vi "Required Buffer Sizes.vi"(8 "error in (no error)":errorcluster, 11 "Transfer Configuration in":refnum<class "Transfer Configuration.lvclass">) -> (0 "error out":errorcluster, 1 "string size":u64 format="%d bytes", 2 "engine size":u64 format="%d bytes", 3 "Transfer Configuration out":refnum<class "Transfer Configuration.lvclass">)   [LabVIEW 2021, in "DSF Core.lvlib" / "Transfer Configuration.lvclass"]
uses:
  Transfer Configuration.lvclass
  Transfer Configuration.lvclass/Transfer Configuration.ctl
  Framework/Framework.lvclass
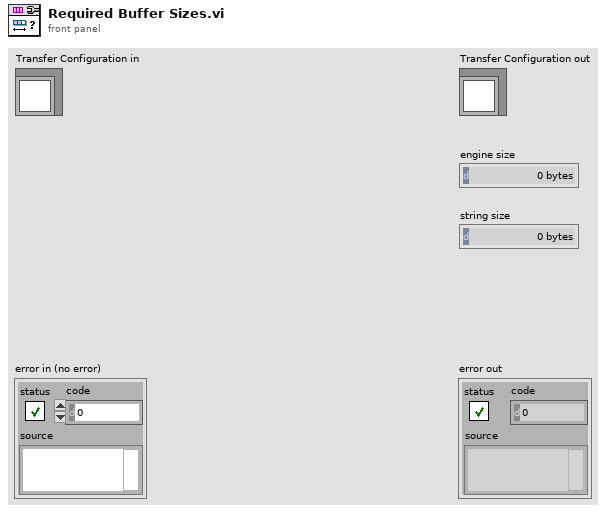
[diagram p1: front panel]
types:
  T1 = typedef "DSF Core.lvlib/Transfer Configuration.lvclass/Channel Configuration.ctl" = cluster{"configuration":T2, "component settings":T4[]}
  T2 = typedef "DSF Core.lvlib/Channel Configuration.lvclass/Core Channel Configuration.ctl" = cluster{"name":string, "units":string, "engine data type":T3, "string data type":T3, "string offset":u64}
  T3 = typedef "DSF Core.lvlib/DSF Data Type.ctl" = enum8{"Bool", "SGL", "DBL", "I8", "I16", "I32", "I64", "U8", "U16", "U32", "U64"}
  T4 = typedef "DSF Core.lvlib/DSF Settings Info.ctl" = cluster{"component":string, "values":cluster{"key":string, "value":string}[]}
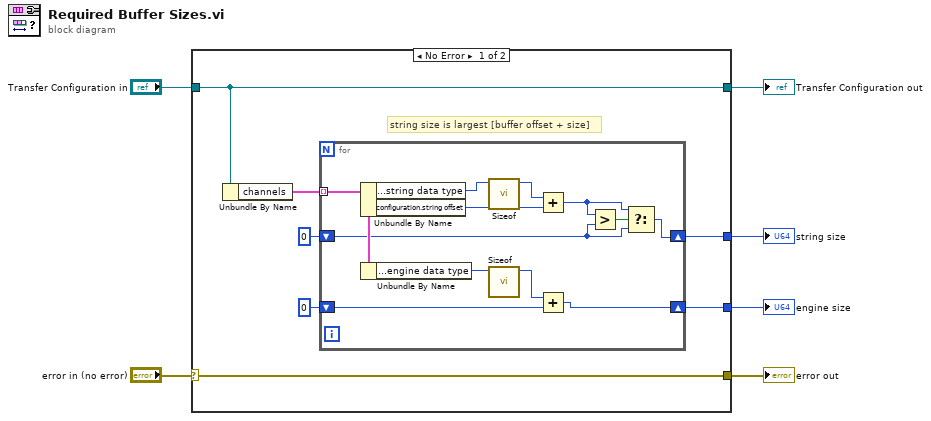
[diagram p0: block diagram]
diagram:
  n1 = case shown="No Error" "error in (no error)" {
    selector: "error in (no error)" -> [w7 w26]
    tunnel: "Transfer Configuration in" -> [w8 w27]
    tunnel: [w10 _] -> w5
    tunnel: [w9 _] -> w4
    tunnel: [w8 w27] -> w3
    tunnel: [w7 w26] -> w1
    frame No Error {
      # "string size is largest [buffer offset + size]"
      n2 = Unbundle By Name(w8) -> ("channels"=w13:T1[])
      n3 = for {
        tunnel: w13 -> [w21] mode=indexing
        shift-right: [w23] -> w10
        shift-left: u64 0 -> [w20]
        shift-right: [w15] -> w9
        shift-left: u64 0 -> [w16]
        n4 = Unbundle By Name(w21) -> ("configuration.string data type"=w19:T3, "configuration.string offset"=w25:u64)
        n5 = Unbundle By Name(w21) -> ("configuration.engine data type"=w17:T3)
        n6 = call "Sizeof.vi"("data type"=w19) -> ("size in bytes"=w18:u64)  [unwired: 9 in, 1 out]
        n7 = call "Sizeof.vi"("data type"=w17) -> ("size in bytes"=w14:u64)  [unwired: 9 in, 1 out]
        n8 = Add(x=w18, y=w25) -> (x+y=w22:u64)
        n9 = Add(x=w14, y=w16) -> (x+y=w15:u64)
        n10 = Greater?(x=w22, y=w20) -> (0:w24:bool)
        n11 = Select(t=w22, s=w24, f=w20) -> (s? t:f=w23:u64)
      }
    }
    frame Error {
    }
  }
  "error out" <- w1
  "Transfer Configuration out" <- w3
  "string size" <- w5
  "engine size" <- w4
